vi "Add File to ProjectItem.vi"(8 "error in (no error)":errorcluster, 10 "File Path":path, 11 "ProjectItem in":refnum<vi>) -> (0 "error out":errorcluster, 2 "Added File ref":refnum<vi>, 3 "ProjectItem out":refnum<vi>)   [LabVIEW 2019, in "gRPC Scripting Tools.lvlib"]
uses:
  gRPC Scripting Tools.lvlib
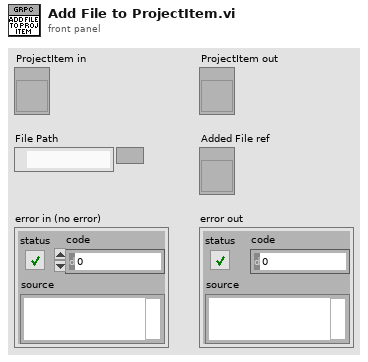
[diagram p1: front panel]
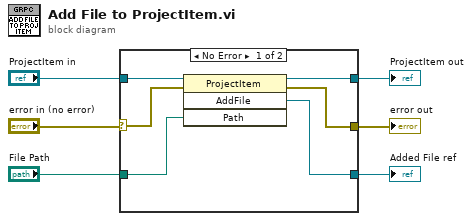
[diagram p0: block diagram]
diagram:
  n1 = case shown="No Error" "error in (no error)" {
    selector: "error in (no error)" -> [w7 w13]
    tunnel: [w12 w13] -> w6
    tunnel: [w11 w14] -> w5
    tunnel: [w10 _] -> w4
    tunnel: "File Path" -> [w9 _]
    tunnel: "ProjectItem in" -> [w8 w14]
    frame No Error {
      n2 = invoke class="ProjectItem" method="AddFile"(reference=w8, error in=w7, "Path"=w9) -> (reference out=w11:refnum<vi>, error out=w12:errorcluster, "AddFile"=w10:refnum<vi>)  [unwired: 1 in, 1 out]
    }
    frame Error {
    }
  }
  "error out" <- w6
  "ProjectItem out" <- w5
  "Added File ref" <- w4
